vi "PR_UW .vi"(8 "error in (no error)":errorcluster, 9 "[workplace_id]":i16=2, 10 "當前工位資料":cluster{"barcode R":string, "barcode L":string}, 11 "DBlink":string="Driver={ODBC Driver 17 for SQL Server};Server=localhost\\SQLEXPRESS;Database=ZDX201;UID=labview;PWD=Dsa@54137926") -> (0 "error out":errorcluster)   [LabVIEW 2019]
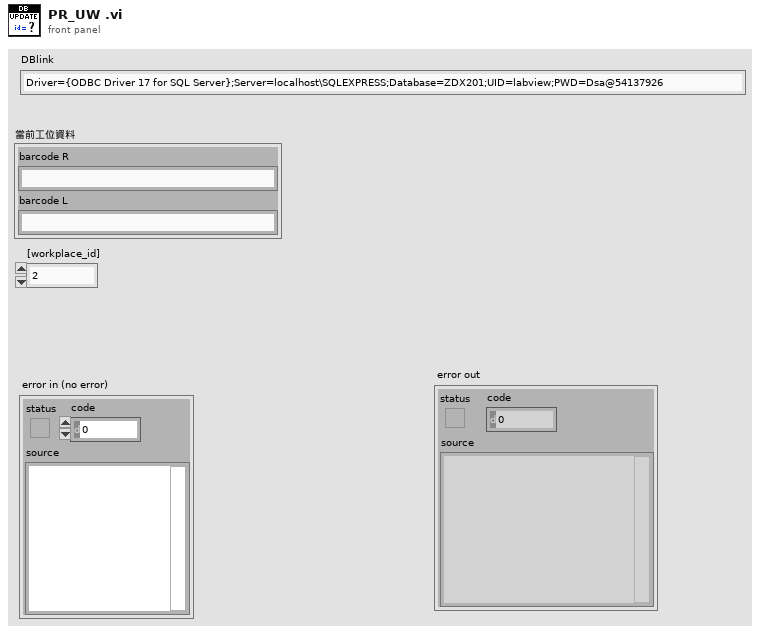
[diagram p1: front panel]
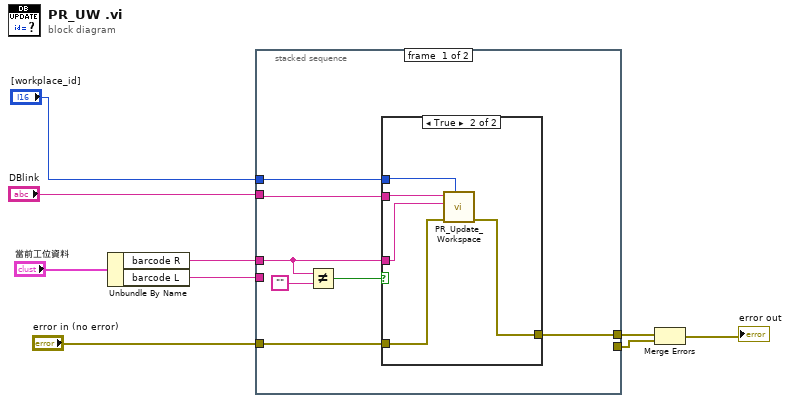
[diagram p0: block diagram]
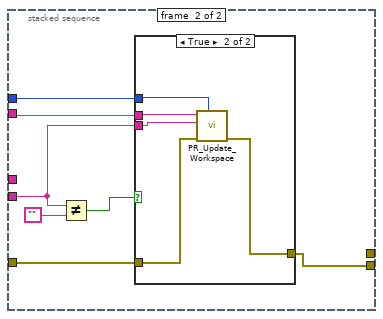
[diagram p3: hidden frame]
diagram:
  n1 = Unbundle By Name("當前工位資料") -> ("barcode R"=w5:string, "barcode L"=w4:string)
  n2 = stacked-sequence {
    tunnel: "[workplace_id]" -> [w16 w29]
    tunnel: "DBlink" -> [w15 w28]
    tunnel: "error in (no error)" -> [w14 w27]
    tunnel: w5 -> [w10 _]
    tunnel: w4 -> [_ w23]
    tunnel: [_ w24] -> w3
    tunnel: [w11 _] -> w2
    frame #0 {
      n3 = Not Equal?(x=w10, y="") -> (x != y?=w12:bool)
      n4 = case shown="True" w12 {
        tunnel: w16 -> [_ w22]
        tunnel: w15 -> [_ w21]
        tunnel: w14 -> [w17 w20]
        tunnel: [w17 w19] -> w11
        tunnel: w10 -> [_ w18]
        frame False {
        }
        frame True {
          n5 = call "PR_Update_Workspace .vi"("[workplace_id]"=w22, "error in (no error)"=w20, "barcode"=w18, "DBlink"=w21) -> ("error out"=w19:errorcluster)  [unwired: 7 in]
        }
      }
    }
    frame #1 {
      n6 = Not Equal?(x=w23, y="") -> (x != y?=w25:bool)
      n7 = case shown="True" w25 {
        tunnel: w29 -> [_ w35]
        tunnel: w28 -> [_ w34]
        tunnel: w27 -> [w30 w33]
        tunnel: [w30 w32] -> w24
        tunnel: w23 -> [_ w31]
        frame False {
        }
        frame True {
          n8 = call "PR_Update_Workspace .vi"("[workplace_id]"=w35, "error in (no error)"=w33, "barcode"=w31, "DBlink"=w34) -> ("error out"=w32:errorcluster)  [unwired: 7 in]
        }
      }
    }
  }
  n9 = Merge Errors(w2, w3) -> (→"error out":errorcluster)
